vi "fpga imaq.vi"   [LabVIEW 2014]
uses:
  <vilib>/visionFPGA/NI_VDM_FPGA_Basics.lvlib
  <vilib>/visionFPGA/Basics/Configure Image Transfer to Target/IMAQ FPGA Configure Image Transfer to Target U8.vi
  <vilib>/visionFPGA/Basics/Image Transfer to Target/IMAQ FPGA Image Transfer to Target U8.vi
  <vilib>/visionFPGA/Basics/Wait for Image Transfer Complete/IMAQ FPGA Wait for Image Transfer Complete U8.vi
  <vilib>/visionFPGA/Basics/Configure Image Transfer from Target/IMAQ FPGA Configure Image Transfer from Target U8.vi
  <vilib>/visionFPGA/Basics/Image Transfer from Target/IMAQ FPGA Image Transfer from Target U8.vi
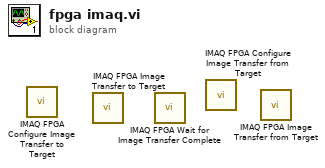
[diagram p0: block diagram]
diagram:
  n1 = call-poly <vilib>:"IMAQ FPGA Configure Image Transfer to Target.vi"() -> ()  [unwired: 8 in, 4 out]
  n2 = call-poly <vilib>:"IMAQ FPGA Image Transfer to Target.vi"() -> ()  [unwired: 9 in, 3 out]
  n3 = call-poly <vilib>:"IMAQ FPGA Wait for Image Transfer Complete.vi"() -> ()  [unwired: 10 in, 2 out]
  n4 = call-poly <vilib>:"IMAQ FPGA Configure Image Transfer from Target.vi"() -> ()  [unwired: 9 in, 3 out]
  n5 = call-poly <vilib>:"IMAQ FPGA Image Transfer from Target.vi"() -> ()  [unwired: 9 in, 3 out]
